vi "Read.vi"(6 "Append Index":i32, 8 "error in (no error)":errorcluster, 11 "Data.TDMS":refnum<class "Data.PG.lvclass">) -> (0 "error out":errorcluster, 1 "Notes":string, 2 "Data (Dictionary)":T1[](array[typedef]), 3 "Data.TDMS out":refnum<class "Data.PG.lvclass">, 5 "Path out":path)   [LabVIEW 2016, in "Data.PG.lvclass"]
uses:
  Data.PG.lvclass
  C:/user/patrick/git/LV-to-ITX/src/Data/Data.lvclass
  Data/Typedefs/Dictionary--cluster.ctl
  <vilib>/JDP Science/PostgreSQL Library/Connection/PQ Connection.lvclass
  Data.PG.lvclass/Data.PG.ctl
  Data/Typedefs/Operation--enum.ctl
  Data/Data.lvclass/Data.ctl
  <vilib>/JDP Science/PostgreSQL Library/Result/PQ Result.lvclass/PQ Result.ctl
  <vilib>/JDP Science/PostgreSQL Library/Connection/Execute Command (2D string results).vi
  <vilib>/JDP Science/PostgreSQL Library/Result/Clear.vi
  <vilib>/JDP Science/PostgreSQL Library/Connection/Execute Command (Result).vi
  <vilib>/JDP Science/PostgreSQL Library/Connection/Execute (Return first result with rows).vi
  <vilib>/JDP Science/PostgreSQL Library/Connection/Single Command with parameters.vi
  <vilib>/JDP Science/PostgreSQL Library/Result/Get all results as 2D strings array.vi
  Data/Data.lvclass
  <vilib>/JDP Science/PostgreSQL Library/Result/PQ Result.lvclass
panel:
  out "size(s)":i32[](array[numeric])
  out "Result":string[][](array[string])
  in  "command":string="SELECT * FROM test_table where my_dbl>0.99;"
  # "MNK"
  # "fsfdfsglkjjjb"
  # "SAMPLE"
  # "GUID EXPT#?"
  # "time"
  # "INST"
  # "ID#"
  # "Vsg"
  # "T"
  # "B"
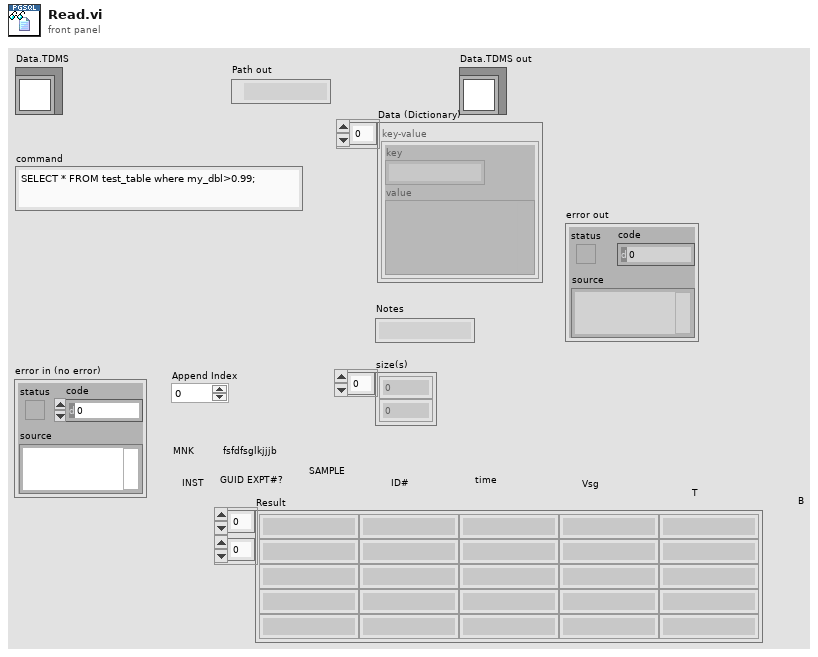
[diagram p1: front panel]
types:
  T1 = typedef "Data.lvclass/Dictionary--cluster.ctl" = cluster{"key":string, "value":variant}
  T2 = typedef "Data.lvclass/Operation--enum.ctl" = enum16{"Read", "Write", "Write + Append"}
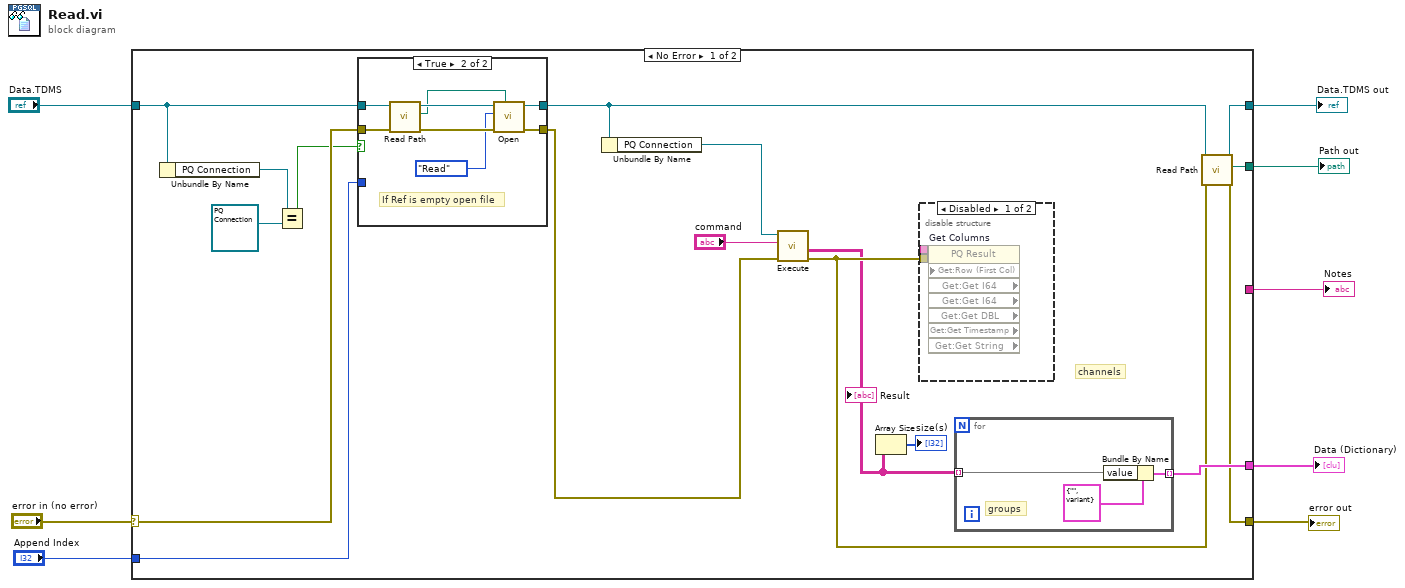
[diagram p0: block diagram]
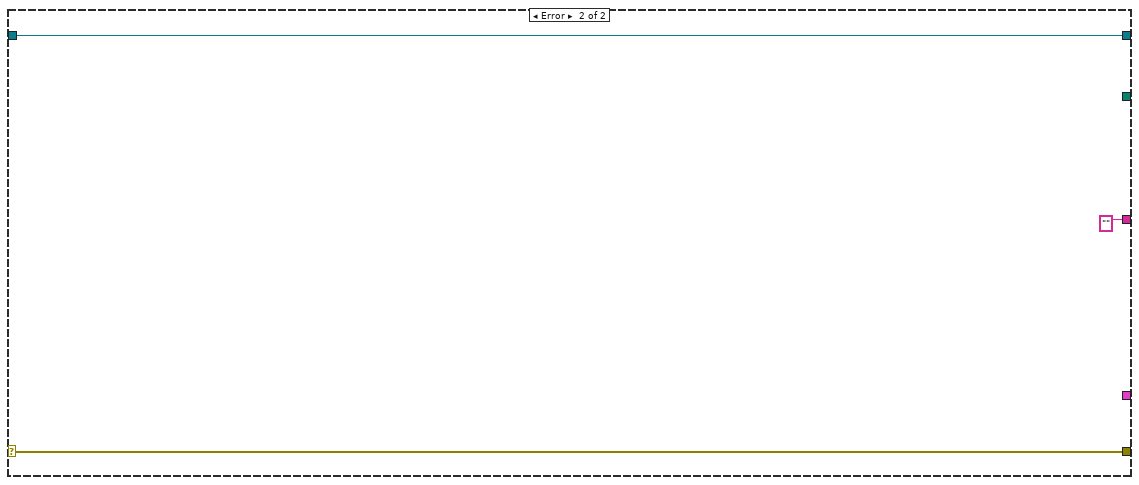
[diagram p4: hidden frame]
diagram:
  n1 = case shown="No Error" "error in (no error)" {
    selector: "error in (no error)" -> [w20 w43]
    tunnel: "Data.TDMS" -> [w21 w42]
    tunnel: [w23 w42] -> w7
    tunnel: [w22 w43] -> w6
    tunnel: [w24 _] -> w5
    tunnel: "Append Index" -> [w16 _]
    tunnel: [w25 _] -> w1
    tunnel: [_ ""] -> w2
    frame No Error {
      # "channels"
      n2 = Unbundle By Name(w21) -> ("PQ Connection"=w18:refnum<class "PQ Connection.lvclass">)
      n3 = Equal?(x=w18, y=refnum<class "PQ Connection.lvclass"> refnum ("PQ Connection")) -> (x = y?=w17:bool)
      n4 = case shown="True" w17 {
        tunnel: w21 -> [w31 w39]
        tunnel: [w31 w40] -> w15
        tunnel: [w32 w36] -> w14
        tunnel: w20 -> [w32 w35]
        tunnel: w16 -> [_ _]
        frame False {
        }
        frame True {
          # "If Ref is empty open file"
          n5 = call "Read Path.vi"("error in (no error)"=w35, "Data Save"=w39) -> ("error out"=w38:errorcluster, "Path"=w34:path, "Data Save out"=w37:refnum<class "Data.PG.lvclass">)  [unwired: 7 in]
          n6 = call-dynamic "Open.vi"("Path"=w34, "error in (no error)"=w38, "Operation"=Operation--enum."Read", "Data.TDMS in"=w37) -> ("error out"=w36:errorcluster, "Data.TDMS out"=w40:refnum<class "Data.PG.lvclass">)  [unwired: 6 in]
        }
      }
      n7 = Unbundle By Name(w15) -> ("PQ Connection"=w12:refnum<class "PQ Connection.lvclass">)
      n8 = call-poly <vilib>:"Execute.vi"("error in (no error)"=w14, "SQL"="command", "PQ Connection in"=w12) -> ("error out"=w11:errorcluster, "Result"=w10:string[][])  [unwired: 5 in, 2 out]
      "Result" <- w10
      n9 = Array Size(array=w10) -> (size(s)=→"size(s)":i32[])
      n10 = disable-structure shown="Disabled" {
        disable-tunnel: _ -> [w30 _]
        disable-tunnel: w11 -> [w29 _]
        frame Disabled {
          n11 = property on="Get Columns" class="PQ Result" props=["Get:Row (First Col)", "Get:Get I64", "Get:Get I64", "Get:Get DBL", "Get:Get Timestamp", "Get:Get String"](reference=w30, error in=w29) -> ()  [unwired: 1 in, 7 out]
        }
        frame Enabled {
        }
      }
      n12 = for {
        tunnel: [w28] -> w25 mode=indexing
        tunnel: w10 -> [w26] mode=indexing
        # "groups"
        n13 = Bundle By Name(cluster=T1 {"key"="", "value"=variant} ("key-value"), "value"=w26) -> (w28:T1)
      }
      n14 = call "Read Path.vi"("error in (no error)"=w11, "Data Save"=w15) -> ("error out"=w22:errorcluster, "Path"=w24:path, "Data Save out"=w23:refnum<class "Data.PG.lvclass">)  [unwired: 7 in]
    }
    frame Error {
    }
  }
  "error out" <- w6
  "Data.TDMS out" <- w7
  "Path out" <- w5
  "Data (Dictionary)" <- w1
  "Notes" <- w2
